vi "AOL Z Cal-Back to normal.vi"   [LabVIEW 2013]
uses:
  Globals/gl_Calibration globals.vi
  Global Variables/gl_UI Ctrl Refs.vi
  Typedefs/Top level VI states.ctl
types:
  T1 = typedef "Top level VI states.ctl" = enum16{"None", "Initialise UI", "<STACK PROTOCOL STATES>", "AOL Zstack-START", "AOL Zstack-STOP", "Motor Zstack-START", "Motor Zstack-STOP", "<ACQUISITION PROTOCOL STATES> ", "Functional Acquisition-START", "Functional Acquisition-STOP", "Single Plane Acquisition-START", "Single Plane Acquisition-STOP", "Volume Acquisition-START", "Volume Acquisition-STOP", "<LIVE IMAGING PROTOCOL STATES>", "Live Imaging-START", "Live Imaging-STOP", "Live Plane Imaging-START", "Live Plane Imaging-STOP", "Live Volume Imaging-START", "Live Volume Imaging-STOP", "EXIT"}
  T2 = typedef "UI ctrl refs cluster.ctl" = cluster{"Top level VI path":path, "Top level VI ref":refnum<vi>, "User menu ref":refnum<k9>, "Sub Panel control":refnum<vi>, "Imaging Param Tab":refnum<vi>, "Occurrence-Start drivers":refnum<k4>, "Occurrence-Speed logging initialised":refnum<k4>, "Occurrence-XYZ stage initialised":refnum<k4>, "Exit button":refnum<vi>, "Status ind":refnum<vi>, "Return to Origin":refnum<vi>, "Speed Logging":refnum<vi>, "Time Lapse":refnum<vi>, "Live Imaging":refnum<vi>, "AOL Z Stack":refnum<vi>, "Motor Z Stack":refnum<vi>, "Funct Acq button":refnum<vi>, "Hard Shutter":refnum<vi>, "Virtual Shutter":refnum<vi>, "Laser Power":refnum<vi>, "AOL Mode":refnum<vi>, "Frame Size":refnum<vi>, "Field of View":refnum<vi>, "Dwell Time":refnum<vi>, "Zoom":refnum<vi>, "AOL Z":refnum<vi>, "Objective":refnum<vi>, "Axis":refnum<vi>, "Paths & Names":refnum<vi>, "Experiment folder path (ind.)":refnum<vi>, "Last State (Ind.)":refnum<vi>, "Laser wavelength ind (nm)":refnum<vi>, "Averages":refnum<vi>, "Angle (degrees)":refnum<vi>, "X centre":refnum<vi>, "Y centre":refnum<vi>, "Plane Mode":refnum<vi>, "# Planes":refnum<vi>, "Z Start":refnum<vi>, "Z Stop":refnum<vi>, "Z Step":refnum<vi>, "PMT 1":refnum<vi>, "PMT 2":refnum<vi>, "Stage XYZ Position":refnum<vi>, "Pockels@Z Start":refnum<vi>, "Pockels@Z Stop":refnum<vi>, "Obtain Z Start":refnum<vi>, "Obtain Z Stop":refnum<vi>, "Live stim.trig.period":refnum<vi>, "Live stim.trig.enable":refnum<vi>, "Funct. Acq. Pockels Modulation":refnum<vi>, "Enable Video Recording":refnum<vi>, "Video Record-Live Imaging":refnum<vi>, "Video Record-Funct acq":refnum<vi>, "AOL Z-stack Chirps Ready (ind)":refnum<vi>, "Center freq ind (nm)":refnum<vi>, "Logging queue (ind)":refnum<vi>, "Back aperture power (ind.)":refnum<vi>, "Power after objective (ind.)":refnum<vi>, "Switch user":refnum<vi>}
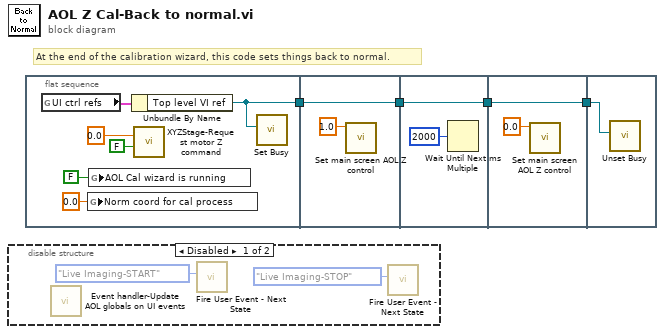
[diagram p0: block diagram]
diagram:
  # "At the end of the calibration wizard, this code sets things back to normal."
  n1 = disable-structure shown="Disabled" {
    frame Disabled {
      n2 = call "Event handler-Update AOL globals on UI events.vi"() -> ()  [unwired: 11 in, 1 out]
      n3 = call "Fire User Event - Next State.vi"("\"UI Handler loop\" case to execute"=Top_level_VI_states."Live Imaging-START" ("\"UI Handler loop\" case to execute")) -> ()  [unwired: 10 in, 1 out]
      n4 = call "Fire User Event - Next State.vi"("\"UI Handler loop\" case to execute"=Top_level_VI_states."Live Imaging-STOP" ("\"UI Handler loop\" case to execute")) -> ()  [unwired: 10 in, 1 out]
    }
    frame Enabled {
    }
  }
  n5 = flat-sequence {
    tunnel: [w11] -> w2
    tunnel: [w14] -> w3
    tunnel: w2 -> [w14]
    tunnel: [w16] -> w4
    tunnel: w3 -> [w16]
    tunnel: [w18] -> w1
    tunnel: w4 -> [w18]
    tunnel: w1 -> [w19]
    frame #0 {
      n6 = global read "gl_UI Ctrl Refs.vi" "UI ctrl refs"() -> (w12:T2)
      n7 = global write "gl_Calibration globals.vi" "Norm coord for cal process"(0.0 ("Norm coord for cal process")) -> ()
      n8 = global write "gl_Calibration globals.vi" "AOL Cal wizard is running"(FALSE ("Motor Z Cal wizard is running")) -> ()
      n9 = Unbundle By Name(w12) -> ("Top level VI ref"=w11:refnum<vi>)
      n10 = call "XYZStage-Request motor Z command.vi"("Wait for acknowledge?"=FALSE, "Motor Z"=sgl 0.0) -> ()  [unwired: 7 in, 3 out]
      n11 = call <vilib>:"Set Busy.vi"("VI reference (current VI)"=w11) -> ()  [unwired: 9 in, 2 out]
    }
    frame #1 {
      n12 = call "Set main screen AOL Z control.vi"("AOL Z Value (Signaling)"=sgl 1.0) -> ()  [unwired: 10 in, 1 out]
    }
    frame #2 {
      n13 = Wait Until Next ms Multiple(millisecond multiple=u32 2000) -> ()  [unwired: 1 out]
    }
    frame #3 {
      n14 = call "Set main screen AOL Z control.vi"("AOL Z Value (Signaling)"=sgl 0.0) -> ()  [unwired: 10 in, 1 out]
    }
    frame #4 {
      n15 = call <vilib>:"Unset Busy.vi"("VI reference (current VI)"=w19) -> ()  [unwired: 10 in, 1 out]
    }
  }
